vi "Write TCPIP address.vi"(8 "error in (no error)":errorcluster, 10 "TCPIP address":refnum<k5>, 11 "ESP301_via_TCPIP in":refnum<class "ESP301_via_TCPIP.lvclass">) -> (0 "error out":errorcluster, 3 "ESP301_via_TCPIP out":refnum<class "ESP301_via_TCPIP.lvclass">)   [LabVIEW 2019, in "ESP301_via_TCPIP.lvclass"]
uses:
  ESP301_via_TCPIP.lvclass
  ESP301_via_TCPIP.lvclass/ESP301_via_TCPIP.ctl
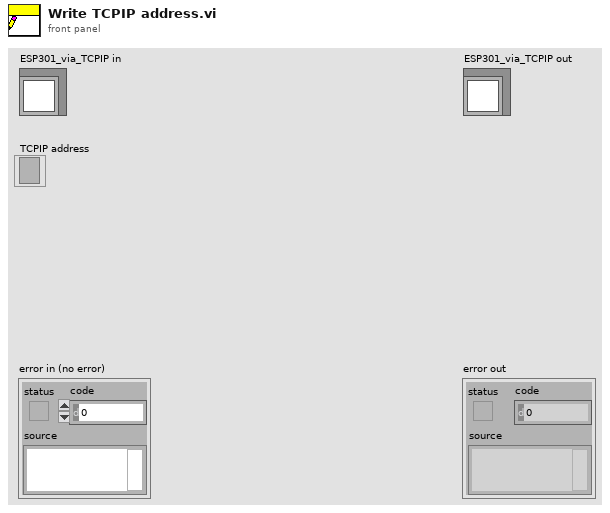
[diagram p1: front panel]
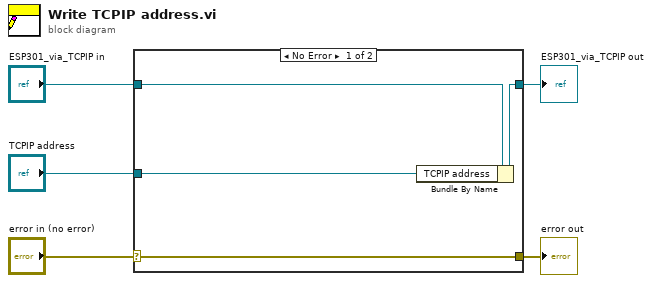
[diagram p0: block diagram]
diagram:
  n1 = case shown="No Error" "error in (no error)" {
    selector: "error in (no error)" -> [w9 w10]
    tunnel: [w9 w10] -> w4
    tunnel: [w7 w11] -> w2
    tunnel: "ESP301_via_TCPIP in" -> [w8 w11]
    tunnel: "TCPIP address" -> [w6 _]
    frame No Error {
      n2 = Bundle By Name(cluster=w8, "TCPIP address"=w6) -> (w7:refnum<class "ESP301_via_TCPIP.lvclass">)
    }
    frame Error {
    }
  }
  "error out" <- w4
  "ESP301_via_TCPIP out" <- w2
